vi "Sample--Sync_MasterSlaveRefClk_PCIe_PCI.vi"() -> ()   [LabVIEW 2013]
doc: "This example demonstrates synchronizing two digitizers."
uses:
  <userlib>/ArtScope/Trigger/ArtScope_ConfigureTriggerDigital.vi
  <userlib>/ArtScope/Fetch/ArtScope_FetchBinary16.vi
  <userlib>/ArtScope/_SubVI/ArtScope_ArrayByChannel_U16.vi
panel:
  out "error out":errorcluster
  in  "reference position2":dbl
  in  "reference position":dbl
  in  "range2(Vpp)":i32(ring) items=["20V", "10V", "2V", "40V", "16V", "8V", "4V", "1.6V", "800m", "400m", "160m", "80m", "40m"]
  in  "range(Vpp)":i32(ring) items=["20V", "10V", "2V", "40V", "16V", "8V", "4V", "1.6V", "800m", "400m", "160m", "80m", "40m"]
  in  "Slave":string="Dev2"
  in  "Master":string="Dev1"
  in  "Stop":bool
  out "Data2":u16[][](graph)
  in  "Timeout(s) 2":dbl=1.0
  in  "MinSampleRate 2":dbl=8000000.0
  in  "MinRecordLength2":i32=6000
  out "Data":u16[][](graph)
  in  "Timeout(s)":dbl=1.0
  in  "MinRecordLength":i32=6000
  in  "MinSampleRate":dbl=8000000.0
  # "Vertical"
  # "Horizontal"
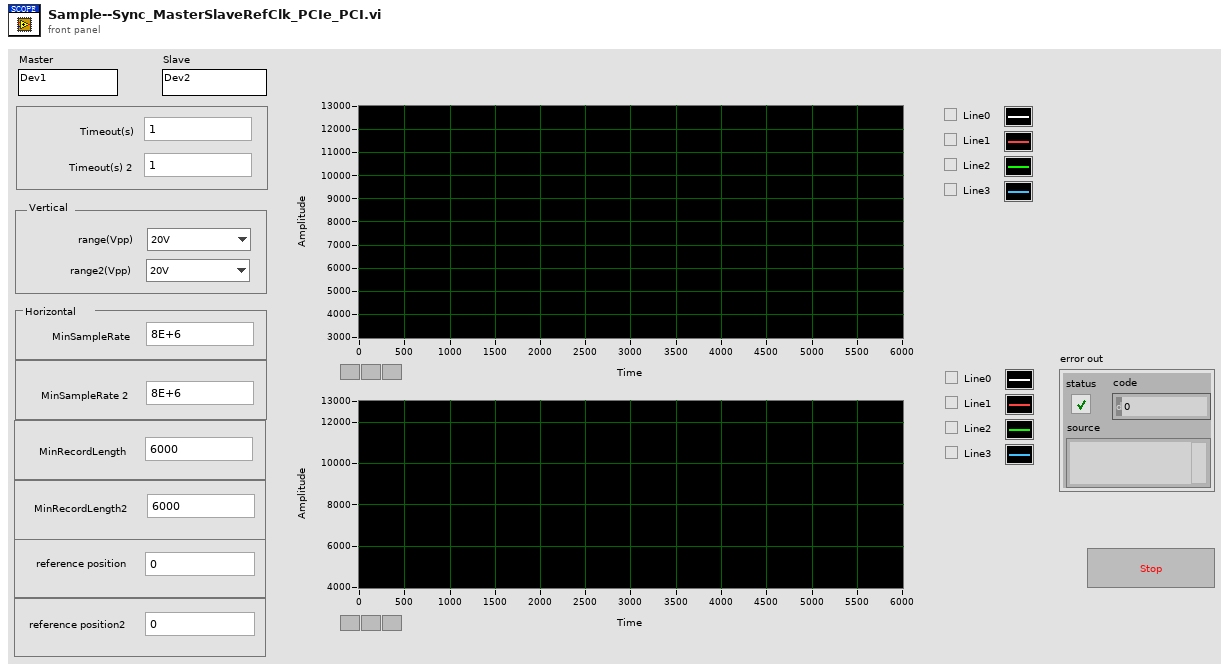
[diagram p1: front panel]
types:
  T1 = cluster{"fLSB":cluster{dbl, dbl, dbl, dbl, dbl, dbl, dbl, dbl}, "RangeValue":cluster{dbl, dbl, dbl, dbl, dbl, dbl, dbl, dbl}, "wMaxLSB":u32, "TriggerMode":i32, "sampLengthPerChan":u32, "pAvailSampsPoints":u32, "channelCount":i32}
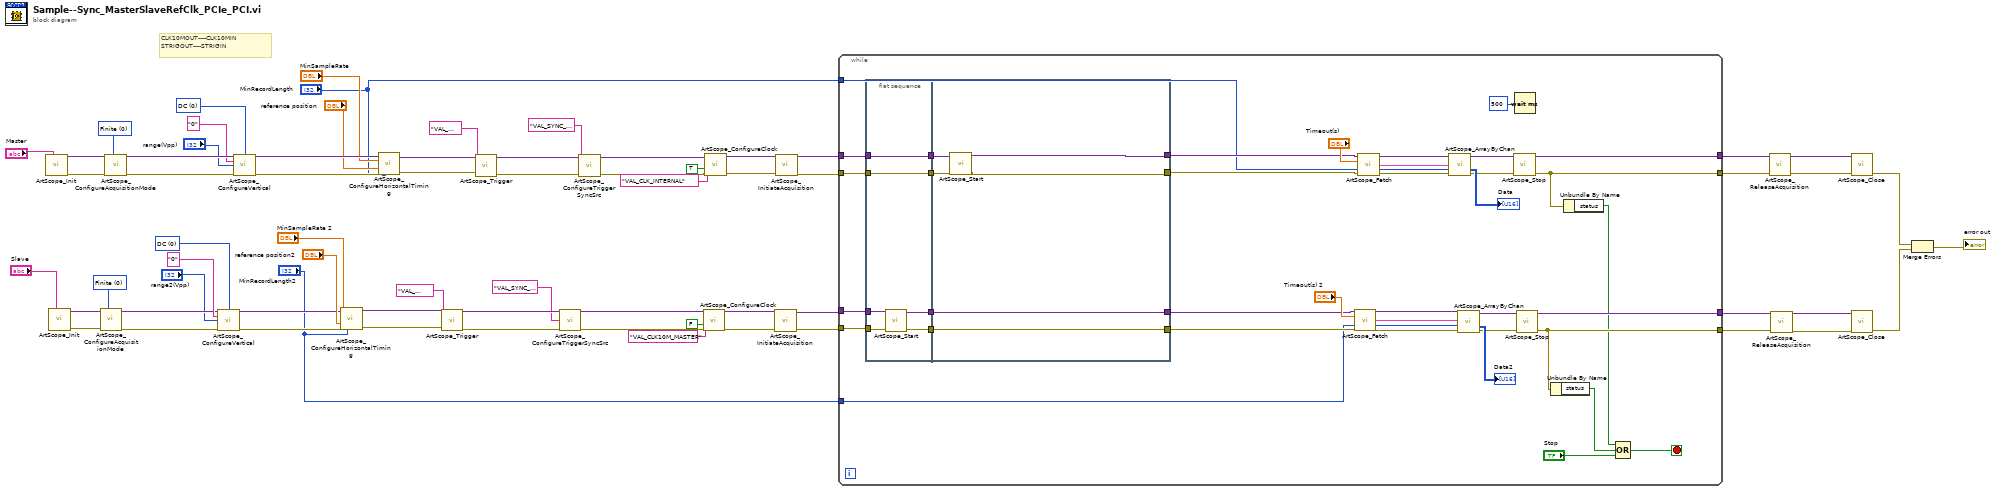
[diagram p0: block diagram]
diagram:
  w50 = 0 items=["DC", "AC"] ("Coupling")
  w56 = 0 items=["Finite", "Continuous"] ("AcuqMode")
  w65 = 0 items=["DC", "AC"] ("Coupling")
  w60 = 0 items=["Finite", "Continuous"] ("AcuqMode")
  # "CLK10MOUT----CLK10MIN\nSTRIGOUT----STRIGIN"
  n1 = call <userlib>:"ArtScope_Init.vi"("task name"="Master") -> ("task handle"=w47:variant, "error out"=w46:errorcluster)  [unwired: 13 in]
  n2 = call <userlib>:"ArtScope_Init.vi"("task name"="Slave") -> ("task handle"=w44:variant, "error out"=w43:errorcluster)  [unwired: 13 in]
  n3 = call <userlib>:"ArtScope_ConfigureAcquisitionMode.vi"("task handle"=w44, "acquisition mode"=w56, "error in (no error)"=w43) -> ("task handle"=w49:variant, "error out"=w48:errorcluster)  [unwired: 11 in]
  n4 = call <userlib>:"ArtScope_ConfigureAcquisitionMode.vi"("task handle"=w47, "acquisition mode"=w60, "error in (no error)"=w46) -> ("task handle"=w59:variant, "error out"=w61:errorcluster)  [unwired: 11 in]
  n5 = call <userlib>:"ArtScope_ConfigureVertical.vi"("task handle"=w49, "coupling"=w50, "channels"="0" ("Channel Name"), "range(Vpp)"="range2(Vpp)", "error in (no error)"=w48) -> ("task handle"=w51:variant, "error out"=w52:errorcluster)  [unwired: 9 in]
  n6 = call <userlib>:"ArtScope_ConfigureVertical.vi"("task handle"=w59, "coupling"=w65, "channels"="0" ("Channel Name"), "range(Vpp)"="range(Vpp)", "error in (no error)"=w61) -> ("task handle"=w64:variant, "error out"=w63:errorcluster)  [unwired: 9 in]
  n7 = call <userlib>:"ArtScope_ConfigureHorizontalTiming.vi"("task handle"=w51, "min sample rate"="MinSampleRate 2", "reference position"="reference position2", "error in (no error)"=w52, "min record length"="MinRecordLength2") -> ("task handle"=w20:variant, "error out"=w19:errorcluster)  [unwired: 9 in]
  n8 = call <userlib>:"ArtScope_ConfigureHorizontalTiming.vi"("task handle"=w64, "min sample rate"="MinSampleRate", "reference position"="reference position", "error in (no error)"=w63, "min record length"="MinRecordLength") -> ("task handle"=w17:variant, "error out"=w16:errorcluster)  [unwired: 9 in]
  n9 = call-poly <userlib>:"ArtScope_Trigger.vi"("task handle"=w20, "trigger source"="VAL_TRIGGER_SYNCTRIGGER", "error in"=w19) -> ("task handle"=w9:variant, "error out"=w7:errorcluster)  [unwired: 11 in]
  n10 = call-poly <userlib>:"ArtScope_Trigger.vi"("task handle"=w17, "trigger source"="VAL_TRIGGER_DTR", "error in"=w16) -> ("task handle"=w13:variant, "error out"=w11:errorcluster)  [unwired: 11 in]
  n11 = call <userlib>:"ArtScope_ConfigureTriggerSyncSrc.vi"("task handle"=w9, "trigger sync source"="VAL_SYNC_TRIGGER0", "error in (no error)"=w7) -> ("task handle"=w8:variant, "error out"=w6:errorcluster)  [unwired: 11 in]
  n12 = call <userlib>:"ArtScope_ConfigureTriggerSyncSrc.vi"("task handle"=w13, "trigger sync source"="VAL_SYNC_TRIGGER0", "error in (no error)"=w11) -> ("task handle"=w12:variant, "error out"=w10:errorcluster)  [unwired: 11 in]
  n13 = call <userlib>:"ArtScope_ConfigureClock.vi"("task handle"=w8, "input clock source"="VAL_CLK10M_MASTER", "master enable"=FALSE, "error in (no error)"=w6) -> ("task handle"=w41:variant, "error out"=w39:errorcluster)  [unwired: 10 in]
  n14 = call <userlib>:"ArtScope_ConfigureClock.vi"("task handle"=w12, "input clock source"="VAL_CLK_INTERNAL", "master enable"=TRUE ("ClkOutEnable"), "error in (no error)"=w10) -> ("task handle"=w35:variant, "error out"=w37:errorcluster)  [unwired: 10 in]
  n15 = call <userlib>:"ArtScope_InitiateAcquisition.vi"("task handle"=w41, "error in (no error)"=w39) -> ("task handle"=w40:variant, "error out"=w38:errorcluster)  [unwired: 12 in]
  n16 = call <userlib>:"ArtScope_InitiateAcquisition.vi"("task handle"=w35, "error in (no error)"=w37) -> ("task handle"=w34:variant, "error out"=w36:errorcluster)  [unwired: 12 in]
  n17 = while {
    tunnel: [w104] -> w33
    tunnel: [w91] -> w31
    tunnel: [w93] -> w29
    tunnel: [w103] -> w26
    tunnel: w40 -> [w102]
    tunnel: w38 -> [w101]
    tunnel: w34 -> [w97]
    tunnel: w36 -> [w96]
    tunnel: "MinRecordLength" -> [w83]
    tunnel: "MinRecordLength2" -> [w82]
    stop <- w88 stop-if-true
    n18 = flat-sequence {
      tunnel: w102 -> [w112]
      tunnel: w101 -> [w111]
      tunnel: [w107] -> w106
      tunnel: [w110] -> w105
      tunnel: [w109] -> w98
      tunnel: w97 -> [w109]
      tunnel: w96 -> [w108]
      tunnel: [w108] -> w95
      tunnel: w106 -> [w118]
      tunnel: w105 -> [w117]
      tunnel: w98 -> [w116]
      tunnel: w95 -> [w115]
      tunnel: [w113] -> w86
      tunnel: [w114] -> w87
      tunnel: [w118] -> w85
      tunnel: [w117] -> w84
      frame #0 {
        n19 = call <userlib>:"ArtScope_Start.vi"("task handle"=w112, "error in (no error)"=w111) -> ("task handle"=w107:variant, "error out"=w110:errorcluster)  [unwired: 12 in]
      }
      frame #1 {
        n20 = call <userlib>:"ArtScope_Start.vi"("task handle"=w116, "error in (no error)"=w115) -> ("task handle"=w114:variant, "error out"=w113:errorcluster)  [unwired: 12 in]
      }
    }
    n21 = call-poly <userlib>:"ArtScope_Fetch.vi"("task handle"=w85, "timeout"="Timeout(s) 2", "num samples"=w82, "error in (no error)"=w84) -> ("task handle"=w73:variant, "wfm info"=w69:T1, "data"=w68:u16[], "error out"=w70:errorcluster)  [unwired: 8 in]
    n22 = call-poly <userlib>:"ArtScope_Fetch.vi"("task handle"=w87, "timeout"="Timeout(s)", "num samples"=w83, "error in (no error)"=w86) -> ("task handle"=w79:variant, "wfm info"=w75:T1, "data"=w74:u16[], "error out"=w78:errorcluster)  [unwired: 8 in]
    n23 = call-poly <userlib>:"ArtScope_ArrayByChan.vi"("task handle"=w79, "wfm info"=w75, "1D data"=w74, "error in (no error)"=w78) -> ("task handle"=w76:variant, "2D data"=→"Data":u16[][], "error out"=w77:errorcluster)  [unwired: 9 in]
    n24 = call-poly <userlib>:"ArtScope_ArrayByChan.vi"("task handle"=w73, "wfm info"=w69, "1D data"=w68, "error in (no error)"=w70) -> ("task handle"=w72:variant, "2D data"=→"Data2":u16[][], "error out"=w71:errorcluster)  [unwired: 9 in]
    n25 = call <userlib>:"ArtScope_Stop.vi"("task handle"=w76, "error in"=w77) -> ("task handle"=w104:variant, "error out"=w91:errorcluster)  [unwired: 12 in]
    n26 = Wait (ms)(milliseconds to wait=u32 500 ("等待时间（毫秒）")) -> ()  [unwired: 1 out]
    n27 = call <userlib>:"ArtScope_Stop.vi"("task handle"=w72, "error in"=w71) -> ("task handle"=w103:variant, "error out"=w93:errorcluster)  [unwired: 12 in]
    n28 = Unbundle By Name(w93) -> ("status"=w92:bool)
    n29 = Unbundle By Name(w91) -> ("status"=w90:bool)
    n30 = Compound Arithmetic op=OR(w90, w92, "Stop") -> (w88:bool)
  }
  n31 = call <userlib>:"ArtScope_ReleaseAcquisition.vi"("task handle"=w33, "error in (no error)"=w31) -> ("task handle"=w32:variant, "error out"=w30:errorcluster)  [unwired: 12 in]
  n32 = call <userlib>:"ArtScope_ReleaseAcquisition.vi"("task handle"=w26, "error in (no error)"=w29) -> ("task handle"=w27:variant, "error out"=w28:errorcluster)  [unwired: 12 in]
  n33 = call <userlib>:"ArtScope_Close.vi"("task handle"=w32, "error in (no error)"=w30) -> ("error out"=w67:errorcluster)  [unwired: 13 in]
  n34 = call <userlib>:"ArtScope_Close.vi"("task handle"=w27, "error in (no error)"=w28) -> ("error out"=w66:errorcluster)  [unwired: 13 in]
  n35 = Merge Errors(w67, w66) -> (→"error out":errorcluster)
